vi "FindInstruments.vi"(8 "error in (no error)":errorcluster, 11 "DongWoo.lvlib:DongWoo.lvclass":refnum<class "DongWoo.lvclass">) -> (0 "error out":errorcluster, 3 "DongWoo.lvlib:DongWoo.lvclass":refnum<class "DongWoo.lvclass">)   [LabVIEW 2023, in "DongWoo_Spectrometer.lvlib" / "DongWoo.lvclass"]
uses:
  DongWoo.lvclass
  DongWoo.lvclass/DongWoo.ctl
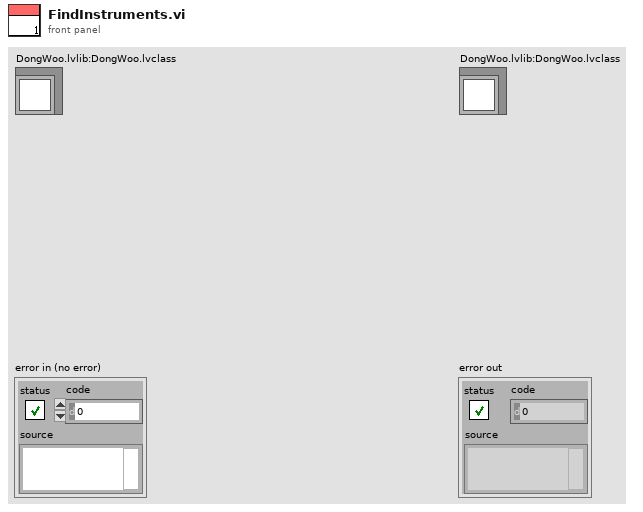
[diagram p1: front panel]
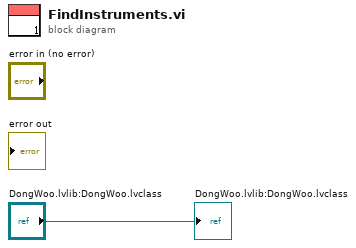
[diagram p0: block diagram]
diagram:
  "DongWoo.lvlib:DongWoo.lvclass" <- "DongWoo.lvlib:DongWoo.lvclass"
